vi "construct_timeout_error.vi"(0 "command in":T1=enum."configure_rf", 11 "error in (no error) 2":errorcluster, 12 "source":string) -> (6 "Multipart message":string[](array[string]), 14 "parameters JSON":string, 15 "error out 2":errorcluster)   [LabVIEW 2019, in "mmW_commands.lvlib"]
uses:
  mmW_commands.lvlib
  TypeDefs/commands.ctl
  TypeDefs/response status.ctl
  typedefs/Response_paramaters.ctl
  typedefs/datatypes_.ctl
  <vilib>/addons/_JKI.lib/Serialization/JSON/JKI JSON Serialization.lvlib
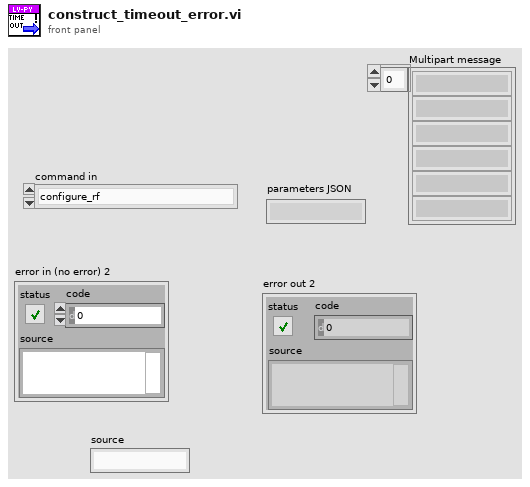
[diagram p1: front panel]
types:
  T1 = typedef "mmW_commands.lvlib/commands.ctl" = enum16{"configure_fs", "configure_rf", "configure_trigger", "equalization_enable", "equalization_start", "lo_sync_enable", "equalization_stop", "get_instrument_status", "get_versions", "initialize_hw", "pop_rx", "set_log_level", "Shutdown", "start", "start_instrument_app", "stop", "trans", "transceive", "trigger_burst", "trigger_sync_enable", "Write TX", "resp_generic", "resp_waveform", "send_trigger", "fetch", "transceive2"}
  T2 = typedef "mmW_commands.lvlib/datatypes_.ctl" = enum16{"none", "string", "interleaved_I16", "interleaved_I32", "I16_array", "I32_array", "JSONstring"}
  T3 = typedef "mmW_commands.lvlib/Response_paramaters.ctl" = cluster{"generic_info":string, "datatype":string, "source":string}
  T4 = typedef "mmW_commands.lvlib/response status.ctl" = enum16{"OK", "Error", "Warning", "Unknown"}
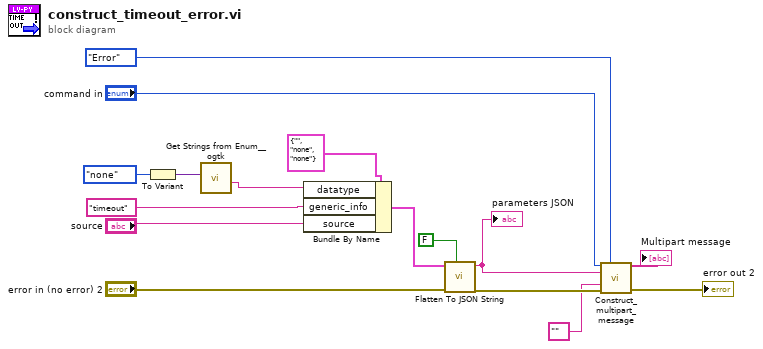
[diagram p0: block diagram]
diagram:
  n1 = To Variant(anything=datatypes_."none" ("datatype")) -> (Variant=w3:variant)
  n2 = call <userlib>:"Get Strings from Enum__ogtk.vi"("Enum"=w3) -> ("String Value"=w1:string)  [unwired: 7 in, 3 out]
  n3 = Bundle By Name(cluster=T3 {"generic_info"="", "datatype"="none", "source"="none"} ("response data"), "datatype"=w1, "generic_info"="timeout", "source"="source") -> (w15:T3)
  n4 = call <vilib>:"Flatten To JSON String.vi"("Multiline (T)"=FALSE, "error in (no error)"="error in (no error) 2", "Variant"=w15) -> ("error out"=w10:errorcluster, "JSON String"=w11:string)  [unwired: 7 in]
  "parameters JSON" <- w11
  n5 = call "Construct_multipart_message.vi"("command"="command in", "Status"=response_status."Error", "parameters (JSON)"=w11, "data in"="", "error in (no error)"=w10) -> ("Multipart message"=→"Multipart message":string[], "error out"=→"error out 2":errorcluster)  [unwired: 7 in, 2 out]
